vi "rad_Get Target Info (IP).vi"(8 "error in (no error)":errorcluster, 11 "Target settings in":T1={"Hostname"="", "Serial number"="", "Product name"="", "Product code"=0, "System status"="", "Credential type"=enum."None/Unlocked", "User added?"=FALSE, "Primary NIC"={"MAC address"="", "IP Address Request Mode"=2, "IP address"="", "Subnet mask"="", "Gateway"="", "DNS server"=""}} {"Primary NIC"."IP Address Request Mode" items=["Static"=1, "DHCP/Link-Local"=2, "Link-Local Only"=4, "DHCP Only"=8]}) -> (0 "error out":errorcluster, 3 "Target settings out":T1={"Hostname"="", "Serial number"="", "Product name"="", "Product code"=0, "System status"="", "Credential type"=enum."None/Unlocked", "User added?"=FALSE, "Primary NIC"={"MAC address"="", "IP Address Request Mode"=2, "IP address"="", "Subnet mask"="", "Gateway"="", "DNS server"=""}} {"Primary NIC"."IP Address Request Mode" items=["Static"=1, "DHCP/Link-Local"=2, "Link-Local Only"=4, "DHCP Only"=8]})   [LabVIEW 2020]
uses:
  support/SubVIs/Target Information.ctl
  TypeDefs/rad_Target Network Settings.ctl
  TypeDefs/rad_Initialize Access Types.ctl
  <vilib>/nisyscfg/Close (System).vi
  <vilib>/nisyscfg/nisyscfg.lvlib
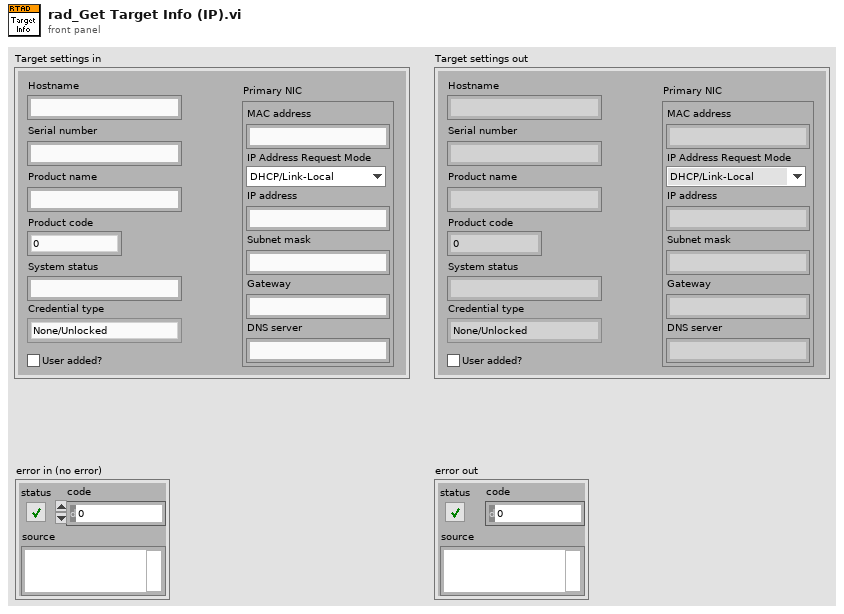
[diagram p1: front panel]
types:
  T1 = typedef "Target Information.ctl" = cluster{"Hostname":string, "Serial number":string, "Product name":string, "Product code":i32, "System status":string, "Credential type":enum16{"None/Unlocked", "FTP Password", "NIAuth Credentials"}, "User added?":bool, "Primary NIC":T2}
  T2 = typedef "rad_Target Network Settings.ctl" = cluster{"MAC address":string, "IP Address Request Mode":i32, "IP address":string, "Subnet mask":string, "Gateway":string, "DNS server":string}
  T3 = typedef "rad_Initialize Access Types.ctl" = enum16{"Anonymous read-only", "Admin unless unlocked", "Admin always"}
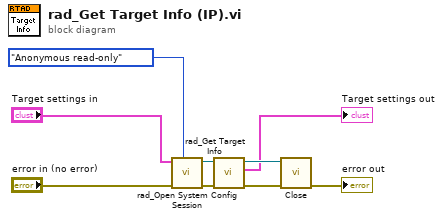
[diagram p0: block diagram]
diagram:
  n1 = call "rad_Open System Config Session.vi"("Access requirement (admin unless unlocked)"=rad_Initialize_Access_Types."Anonymous read-only", "error in (no error)"="error in (no error)", "Target settings"="Target settings in") -> ("error out"=w5:errorcluster, "Session out"=w4:refnum<k21>)  [unwired: 5 in, 2 out]
  n2 = call "rad_Get Target Info.vi"("error in (no error)"=w5, "System Session in"=w4) -> ("error out"=w6:errorcluster, "Target settings"=→"Target settings out":T1, "System Session out"=w7:refnum<k21>)  [unwired: 7 in]
  n3 = call-poly <vilib>:"Close.vi"("error in (no error)"=w6, "Session in"=w7) -> ("error out"=→"error out":errorcluster)  [unwired: 9 in]
